vi "Configuration Convert 1.2 to 1.1.vi"(8 "error in (no error)":errorcluster, 11 "configuration 1.2":T2={"plugins"=[{"name"="", "components"=[], "cycle timing"={"priority"=100, "decimation"=1, "offset"=0}, "threads"=[{"processor"=-2, "priority offset"=0, "settings"=[]}, {"processor"=-2, "priority offset"=0, "settings"=[]}, {"processor"=-2, "priority offset"=0, "settings"=[]}, {"processor"=-2, "priority offset"=0, "settings"=[]}], "transfer groups"=[{"name"="", "direction"=enum."Tx", "cycle timing"={"priority"=100, "decimation"=1, "offset"=0}, "thread index"=0, "settings"=[], "transfers"=[{"name"="", "byte order"=enum."big-endian", "settings"=[], "channels"=[]}], "timeout behavior"=enum."Increment Late Count"}], "settings"=[]}]}) -> (0 "error out":errorcluster, 3 "configuration 1.1":T1={"plugins"=[{"name"="Plugin", "components"=[], "cycle timing"={"priority"=10000, "decimation"=1, "offset"=0}, "threads"=[], "transfer groups"=[{"name"="Group", "direction"=0, "cycle timing"={"priority"=100, "decimation"=1, "offset"=0}, "thread index"=-1, "settings"=[], "transfers"=[{"name"="Transfer", "byte order"=0, "settings"=[], "channels"=[{"string offset"=0, "string data type"=2, "engine data type"=2, "name"="Channel", "settings"=[], "units"="V"}]}], "timeout behavior"=0}], "settings"=[]}]})   [LabVIEW 2017, in "DSF Core.lvlib" / "Configuration Session.lvclass"]
uses:
  Configuration Session.lvclass
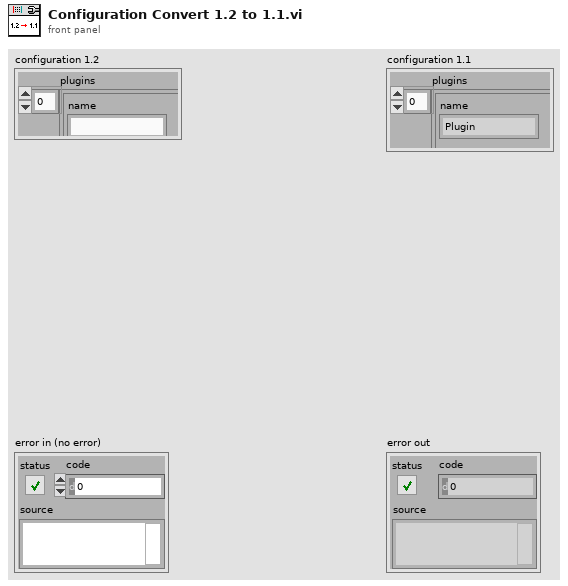
[diagram p1: front panel]
types:
  T1 = cluster{"plugins":cluster{"name":string, "components":string[], "cycle timing":cluster{"priority":u64, "decimation":u64, "offset":u64}, "threads":cluster{"buffer converter settings":cluster{"key":string, "value":string}[], "transceiver settings":cluster{"key":string, "value":string}[], "custom settings":cluster{"key":string, "value":string}[], "processor":i32, "priority offset":i16}[], "transfer groups":cluster{"name":string, "direction":u8, "cycle timing":cluster{"priority":u64, "decimation":u64, "offset":u64}, "thread index":i32, "settings":cluster{"key":string, "value":string}[], "transfers":cluster{"name":string, "byte order":u8, "settings":cluster{"key":string, "value":string}[], "channels":cluster{"string offset":u64, "string data type":u8, "engine data type":u8, "name":string, "settings":cluster{"key":string, "value":string}[], "units":string}[]}[], "timeout behavior":u8}[], "settings":cluster{"key":string, "value":string}[]}[]}
  T2 = cluster{"plugins":cluster{"name":string, "components":string[], "cycle timing":cluster{"priority":u64, "decimation":u64, "offset":u64}, "threads":cluster{"processor":i32, "priority offset":i16, "settings":cluster{"component":string, "name":string, "values":cluster{"key":string, "value":string}[]}[]}[], "transfer groups":cluster{"name":string, "direction":enum8{"Tx", "Rx"}, "cycle timing":cluster{"priority":u64, "decimation":u64, "offset":u64}, "thread index":i32, "settings":cluster{"component":string, "name":string, "values":cluster{"key":string, "value":string}[]}[], "transfers":cluster{"name":string, "byte order":enum8{"big-endian", "little-endian"}, "settings":cluster{"component":string, "name":string, "values":cluster{"key":string, "value":string}[]}[], "channels":cluster{"string offset":u64, "name":string, "units":string, "engine data type":enum8{"Bool", "SGL", "DBL", "I8", "I16", "I32", "I64", "U8", "U16", "U32", "U64"}, "string data type":enum8{"Bool", "SGL", "DBL", "I8", "I16", "I32", "I64", "U8", "U16", "U32", "U64"}, "settings":cluster{"component":string, "name":string, "values":cluster{"key":string, "value":string}[]}[]}[]}[], "timeout behavior":enum8{"Increment Late Count", "Throw Error"}}[], "settings":cluster{"component":string, "name":string, "values":cluster{"key":string, "value":string}[]}[]}[]}
  T3 = cluster{"name":string, "components":string[], "cycle timing":cluster{"priority":u64, "decimation":u64, "offset":u64}, "threads":cluster{"buffer converter settings":cluster{"key":string, "value":string}[], "transceiver settings":cluster{"key":string, "value":string}[], "custom settings":cluster{"key":string, "value":string}[], "processor":i32, "priority offset":i16}[], "transfer groups":cluster{"name":string, "direction":u8, "cycle timing":cluster{"priority":u64, "decimation":u64, "offset":u64}, "thread index":i32, "settings":cluster{"key":string, "value":string}[], "transfers":cluster{"name":string, "byte order":u8, "settings":cluster{"key":string, "value":string}[], "channels":cluster{"string offset":u64, "string data type":u8, "engine data type":u8, "name":string, "settings":cluster{"key":string, "value":string}[], "units":string}[]}[], "timeout behavior":u8}[], "settings":cluster{"key":string, "value":string}[]}
  T4 = cluster{"name":string, "direction":u8, "cycle timing":cluster{"priority":u64, "decimation":u64, "offset":u64}, "thread index":i32, "settings":cluster{"key":string, "value":string}[], "transfers":cluster{"name":string, "byte order":u8, "settings":cluster{"key":string, "value":string}[], "channels":cluster{"string offset":u64, "string data type":u8, "engine data type":u8, "name":string, "settings":cluster{"key":string, "value":string}[], "units":string}[]}[], "timeout behavior":u8}
  T5 = cluster{"name":string, "byte order":u8, "settings":cluster{"key":string, "value":string}[], "channels":cluster{"string offset":u64, "string data type":u8, "engine data type":u8, "name":string, "settings":cluster{"key":string, "value":string}[], "units":string}[]}
  T6 = cluster{"string offset":u64, "string data type":u8, "engine data type":u8, "name":string, "settings":cluster{"key":string, "value":string}[], "units":string}
  T7 = cluster{"buffer converter settings":cluster{"key":string, "value":string}[], "transceiver settings":cluster{"key":string, "value":string}[], "custom settings":cluster{"key":string, "value":string}[], "processor":i32, "priority offset":i16}
  T8 = cluster{"name":string, "components":string[], "cycle timing":cluster{"priority":u64, "decimation":u64, "offset":u64}, "threads":cluster{"processor":i32, "priority offset":i16, "settings":cluster{"component":string, "name":string, "values":cluster{"key":string, "value":string}[]}[]}[], "transfer groups":cluster{"name":string, "direction":enum8{"Tx", "Rx"}, "cycle timing":cluster{"priority":u64, "decimation":u64, "offset":u64}, "thread index":i32, "settings":cluster{"component":string, "name":string, "values":cluster{"key":string, "value":string}[]}[], "transfers":cluster{"name":string, "byte order":enum8{"big-endian", "little-endian"}, "settings":cluster{"component":string, "name":string, "values":cluster{"key":string, "value":string}[]}[], "channels":cluster{"string offset":u64, "name":string, "units":string, "engine data type":enum8{"Bool", "SGL", "DBL", "I8", "I16", "I32", "I64", "U8", "U16", "U32", "U64"}, "string data type":enum8{"Bool", "SGL", "DBL", "I8", "I16", "I32", "I64", "U8", "U16", "U32", "U64"}, "settings":cluster{"component":string, "name":string, "values":cluster{"key":string, "value":string}[]}[]}[]}[], "timeout behavior":enum8{"Increment Late Count", "Throw Error"}}[], "settings":cluster{"component":string, "name":string, "values":cluster{"key":string, "value":string}[]}[]}[]
  T9 = cluster{"priority":u64, "decimation":u64, "offset":u64}
  T10 = cluster{"component":string, "name":string, "values":cluster{"key":string, "value":string}[]}[]
  T11 = cluster{"processor":i32, "priority offset":i16, "settings":cluster{"component":string, "name":string, "values":cluster{"key":string, "value":string}[]}[]}[]
  T12 = cluster{"name":string, "direction":enum8{"Tx", "Rx"}, "cycle timing":cluster{"priority":u64, "decimation":u64, "offset":u64}, "thread index":i32, "settings":cluster{"component":string, "name":string, "values":cluster{"key":string, "value":string}[]}[], "transfers":cluster{"name":string, "byte order":enum8{"big-endian", "little-endian"}, "settings":cluster{"component":string, "name":string, "values":cluster{"key":string, "value":string}[]}[], "channels":cluster{"string offset":u64, "name":string, "units":string, "engine data type":enum8{"Bool", "SGL", "DBL", "I8", "I16", "I32", "I64", "U8", "U16", "U32", "U64"}, "string data type":enum8{"Bool", "SGL", "DBL", "I8", "I16", "I32", "I64", "U8", "U16", "U32", "U64"}, "settings":cluster{"component":string, "name":string, "values":cluster{"key":string, "value":string}[]}[]}[]}[], "timeout behavior":enum8{"Increment Late Count", "Throw Error"}}[]
  T13 = cluster{"name":string, "byte order":enum8{"big-endian", "little-endian"}, "settings":cluster{"component":string, "name":string, "values":cluster{"key":string, "value":string}[]}[], "channels":cluster{"string offset":u64, "name":string, "units":string, "engine data type":enum8{"Bool", "SGL", "DBL", "I8", "I16", "I32", "I64", "U8", "U16", "U32", "U64"}, "string data type":enum8{"Bool", "SGL", "DBL", "I8", "I16", "I32", "I64", "U8", "U16", "U32", "U64"}, "settings":cluster{"component":string, "name":string, "values":cluster{"key":string, "value":string}[]}[]}[]}[]
  T14 = cluster{"string offset":u64, "name":string, "units":string, "engine data type":enum8{"Bool", "SGL", "DBL", "I8", "I16", "I32", "I64", "U8", "U16", "U32", "U64"}, "string data type":enum8{"Bool", "SGL", "DBL", "I8", "I16", "I32", "I64", "U8", "U16", "U32", "U64"}, "settings":cluster{"component":string, "name":string, "values":cluster{"key":string, "value":string}[]}[]}[]
  T15 = enum8{"Bool", "SGL", "DBL", "I8", "I16", "I32", "I64", "U8", "U16", "U32", "U64"}
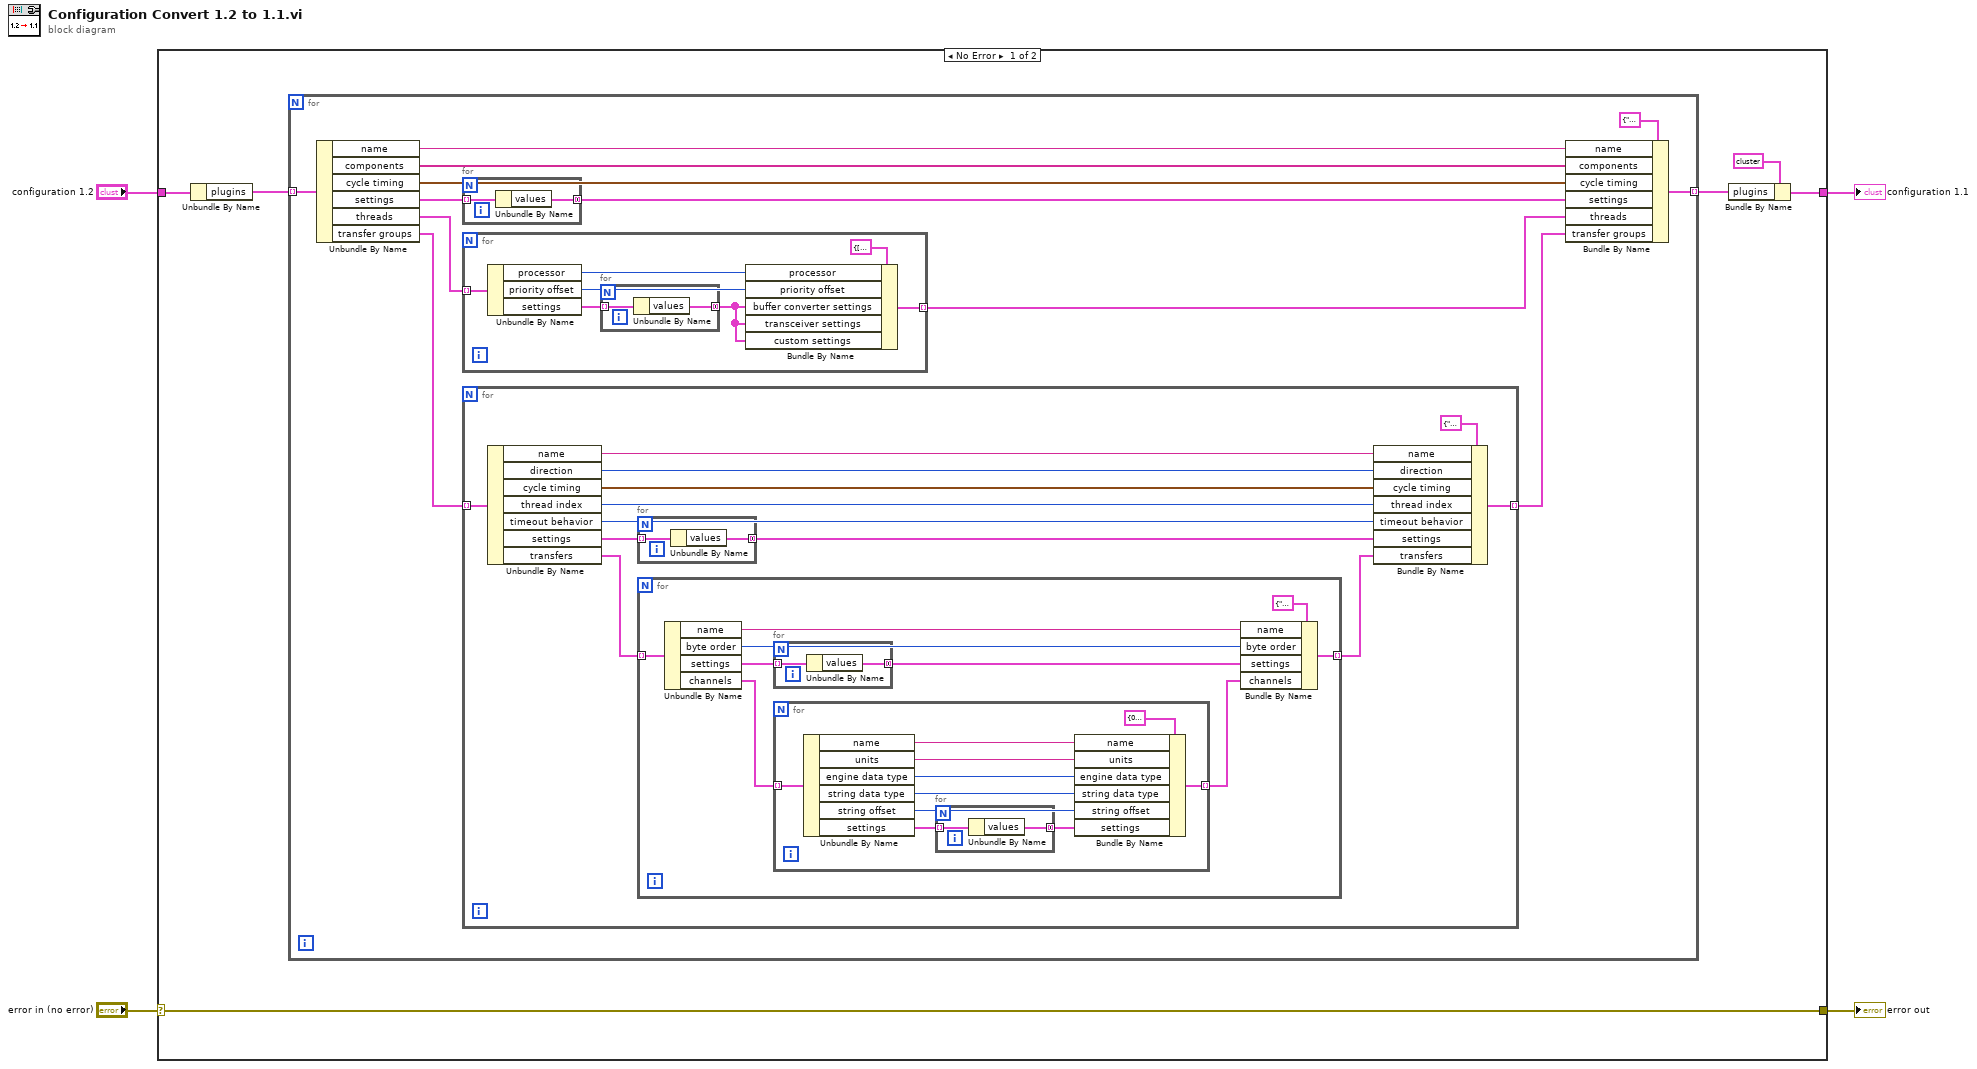
[diagram p0: block diagram]
diagram:
  n1 = case shown="No Error" "error in (no error)" {
    selector: "error in (no error)" -> [w10 w71]
    tunnel: [w10 w71] -> w4
    tunnel: "configuration 1.2" -> [w9 _]
    tunnel: [w7 _] -> w1
    frame No Error {
      n2 = Unbundle By Name(w9) -> ("plugins"=w6:T8)
      n3 = for {
        tunnel: w6 -> [w20] mode=indexing
        tunnel: [w21] -> w5 mode=indexing
        n4 = Unbundle By Name(w20) -> ("name"=w19:string, "components"=w18:string[], "cycle timing"=w17:T9, "settings"=w16:T10, "threads"=w14:T11, "transfer groups"=w12:T12)
        n5 = for {
          tunnel: w16 -> [w70] mode=indexing
          tunnel: [w69] -> w15 mode=concatenating
          n6 = Unbundle By Name(w70) -> ("values"=w69:cluster{"key":string, "value":string}[])
        }
        n7 = for {
          tunnel: w14 -> [w66] mode=indexing
          tunnel: [w60] -> w13 mode=indexing
          n8 = Unbundle By Name(w66) -> ("processor"=w63:i32, "priority offset"=w62:i16, "settings"=w65:T10)
          n9 = for {
            tunnel: w65 -> [w68] mode=indexing
            tunnel: [w67] -> w61 mode=concatenating
            n10 = Unbundle By Name(w68) -> ("values"=w67:cluster{"key":string, "value":string}[])
          }
          n11 = Bundle By Name(cluster=T7 {"buffer converter settings"=[], "transceiver settings"=[], "custom settings"=[], "processor"=0, "priority offset"=0} ("threads"), "processor"=w63, "priority offset"=w62, "buffer converter settings"=w61, "transceiver settings"=w61, "custom settings"=w61) -> (w60:T7)
        }
        n12 = for {
          tunnel: w12 -> [w33] mode=indexing
          tunnel: [w31] -> w11 mode=indexing
          n13 = Unbundle By Name(w33) -> ("name"=w32:string, "direction"=w30:enum8{"Tx", "Rx"}, "cycle timing"=w29:T9, "thread index"=w28:i32, "timeout behavior"=w27:enum8{"Increment Late Count", "Throw Error"}, "settings"=w26:T10, "transfers"=w24:T13)
          n14 = for {
            tunnel: w26 -> [w59] mode=indexing
            tunnel: [w58] -> w25 mode=concatenating
            n15 = Unbundle By Name(w59) -> ("values"=w58:cluster{"key":string, "value":string}[])
          }
          n16 = for {
            tunnel: w24 -> [w42] mode=indexing
            tunnel: [w39] -> w23 mode=indexing
            n17 = Unbundle By Name(w42) -> ("name"=w41:string, "byte order"=w40:enum8{"big-endian", "little-endian"}, "settings"=w38:T10, "channels"=w36:T14)
            n18 = for {
              tunnel: w38 -> [w57] mode=indexing
              tunnel: [w56] -> w37 mode=concatenating
              n19 = Unbundle By Name(w57) -> ("values"=w56:cluster{"key":string, "value":string}[])
            }
            n20 = for {
              tunnel: w36 -> [w53] mode=indexing
              tunnel: [w46] -> w35 mode=indexing
              n21 = Unbundle By Name(w53) -> ("name"=w51:string, "units"=w50:string, "engine data type"=w49:T15, "string data type"=w48:T15, "string offset"=w47:u64, "settings"=w45:T10)
              n22 = for {
                tunnel: w45 -> [w55] mode=indexing
                tunnel: [w54] -> w44 mode=concatenating
                n23 = Unbundle By Name(w55) -> ("values"=w54:cluster{"key":string, "value":string}[])
              }
              n24 = Bundle By Name(cluster=T6 {"string offset"=0, "string data type"=0, "engine data type"=0, "name"="", "settings"=[], "units"=""} ("channels"), "name"=w51, "units"=w50, "engine data type"=w49, "string data type"=w48, "string offset"=w47, "settings"=w44) -> (w46:T6)
            }
            n25 = Bundle By Name(cluster=T5 {"name"="", "byte order"=0, "settings"=[], "channels"=[]} ("transfers"), "name"=w41, "byte order"=w40, "settings"=w37, "channels"=w35) -> (w39:T5)
          }
          n26 = Bundle By Name(cluster=T4 {"name"="", "direction"=0, "cycle timing"={"priority"=0, "decimation"=0, "offset"=0}, "thread index"=0, "settings"=[], "transfers"=[], "timeout behavior"=0} ("transfer groups"), "name"=w32, "direction"=w30, "cycle timing"=w29, "thread index"=w28, "timeout behavior"=w27, "settings"=w25, "transfers"=w23) -> (w31:T4)
        }
        n27 = Bundle By Name(cluster=T3 {"name"="", "components"=[], "cycle timing"={"priority"=0, "decimation"=0, "offset"=0}, "threads"=[], "transfer groups"=[], "settings"=[]} ("plugins"), "name"=w19, "components"=w18, "cycle timing"=w17, "settings"=w15, "threads"=w13, "transfer groups"=w11) -> (w21:T3)
      }
      n28 = Bundle By Name(cluster=T1 {"plugins"=[{"name"="Plugin", "components"=[], "cycle timing"={"priority"=10000, "decimation"=1, "offset"=0}, "threads"=[], "transfer groups"=[{"name"="Group", "direction"=0, "cycle timing"={"priority"=100, "decimation"=1, "offset"=0}, "thread index"=-1, "settings"=[], "transfers"=[{"name"="Transfer", "byte order"=0, "settings"=[], "channels"=[{"string offset"=0, "string data type"=2, "engine data type"=2, "name"="Channel", "settings"=[], "units"="V"}]}], "timeout behavior"=0}], "settings"=[]}]} ("configuration 1.1"), "plugins"=w5) -> (w7:T1)
    }
    frame Error {
    }
  }
  "error out" <- w4
  "configuration 1.1" <- w1
